vi "Export to JSON RTM.vi"(8 "error in":errorcluster, 11 "Node Ptr":u64 format="%.0x") -> (0 "error out":errorcluster)   [LabVIEW 2026, in "Template System Explorer.lvlib"]
uses:
  Template System Explorer.lvlib
  NationalInstruments.VeriStand.SystemDefinitionAPI
panel:
  in  "Tag":string
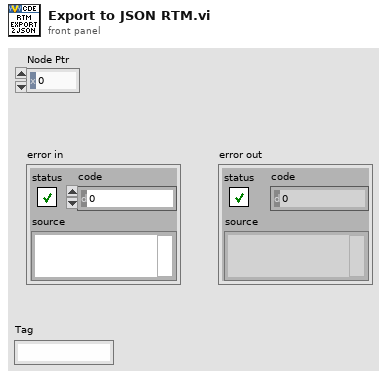
[diagram p1: front panel]
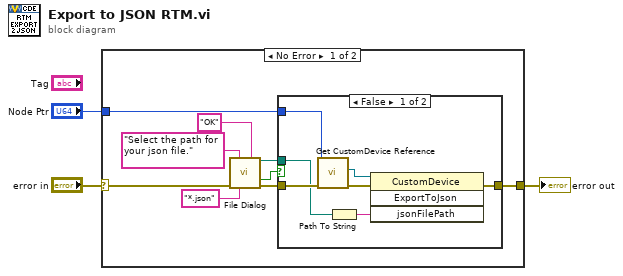
[diagram p0: block diagram]
diagram:
  n1 = case shown="No Error" "error in" {
    selector: "error in" -> [w12 w21]
    tunnel: [w11 w21] -> w1
    tunnel: "Node Ptr" -> [w10 _]
    frame No Error {
      n2 = call "File Dialog"("prompt"="Select the path for your json file.", "button label"="OK", "error in"=w12, "pattern (all files)"="*.json") -> ("selected path"=w7:path, "cancelled"=w4:bool, "error out"=w6:errorcluster)  [unwired: 8 in, 1 out]
      n3 = case shown="False" w4 {
        tunnel: w7 -> [w18 _]
        tunnel: w6 -> [w19 w20]
        tunnel: [w17 w20] -> w11
        tunnel: w10 -> [w16 _]
        frame False {
          n4 = call "Get CustomDevice Reference.vi"("error in"=w19, "Node Ptr"=w16) -> ("error out"=w14:errorcluster, "Custom Device"=w13:refnum<k24>)  [unwired: 7 in, 1 out]
          n5 = Path To String(path=w18) -> (string=w15:string)
          n6 = invoke class="CustomDevice" method="ExportToJson"(reference=w13, error in=w14, "jsonFilePath"=w15) -> (error out=w17:errorcluster)  [unwired: 1 in, 3 out]
        }
        frame True {
        }
      }
    }
    frame Error {
    }
  }
  "error out" <- w1
